vi "Check.vi"(8 "error in (no error)":errorcluster, 11 "Blacklist in":refnum<class "Blacklist.lvclass">) -> (0 "error out":errorcluster, 1 "Reject?":bool, 2 "Output":string, 3 "Blacklist out":refnum<class "Blacklist.lvclass">)   [LabVIEW 2014, in "BuildSecurity.lvlib" / "Blacklist.lvclass"]
doc: "Checks if a VI contains a blacklisted item. If an item is found, <b>Reject?</b> will return <b>TRUE</b>."
uses:
  Blacklist.lvclass
  <vilib>/Utility/traverseref.llb/TRef TravTarget.ctl
  Blacklist.lvclass/Blacklist.ctl
  <vilib>/Utility/traverseref.llb/VI Scripting - Traverse.lvlib
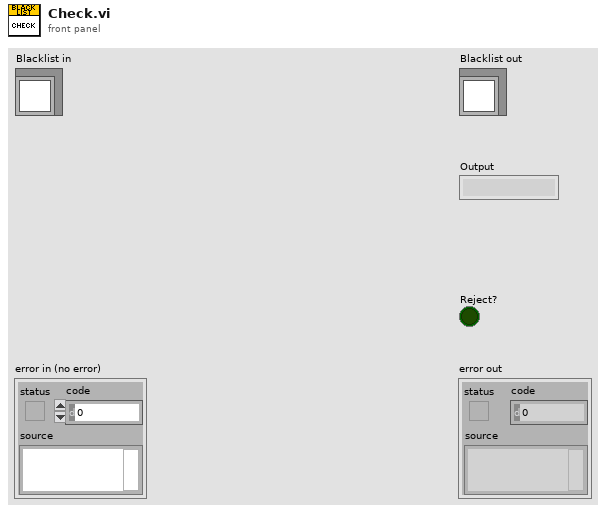
[diagram p1: front panel]
types:
  T1 = typedef "TRef TravTarget.ctl" = enum16{"FP", "BD", "Other"}
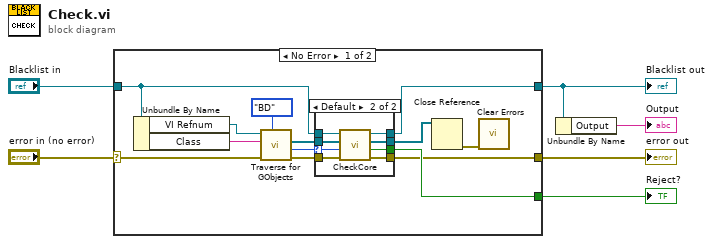
[diagram p0: block diagram]
diagram:
  n1 = case shown="No Error" "error in (no error)" {
    selector: "error in (no error)" -> [w18 w32]
    tunnel: [w7 w32] -> w5
    tunnel: [w11 w31] -> w2
    tunnel: "Blacklist in" -> [w12 w31]
    tunnel: [w9 _] -> w3
    frame No Error {
      n2 = Unbundle By Name(w12) -> ("VI Refnum"=w16:refnum<vi>, "Class"=w19:string)
      n3 = call <vilib>:"Traverse for GObjects.vi"("Traverse Target"=TRef_TravTarget."BD", "error in (no error)"=w18, "Class Name"=w19, "VI Refnum"=w16) -> ("error out"=w14:errorcluster, "# of Refs"=w15:i32, "References"=w13:refnum<vi>[])  [unwired: 4 in, 1 out]
      n4 = case shown="Default" w15 {
        selector: w15 -> [_ w27]
        tunnel: w14 -> [w20 w30]
        tunnel: w13 -> [w21 w28]
        tunnel: w12 -> [w22 w29]
        tunnel: [w22 w26] -> w11
        tunnel: [w21 w25] -> w10
        tunnel: [_ w24] -> w9
        tunnel: [w20 w23] -> w7
        frame 0 {
        }
        frame Default {
          n5 = call-dynamic "CheckCore.vi"("error in (no error)"=w30, "# of Refs"=w27, "References"=w28, "Blacklist in"=w29) -> ("error out"=w23:errorcluster, "Reject?"=w24:bool, "dup References"=w25:refnum<vi>[], "Blacklist out"=w26:refnum<class "Blacklist.lvclass">)  [unwired: 4 in]
        }
      }
      n6 = Close Reference(reference=w10) -> (error out=w8:errorcluster)  [unwired: 1 in]
      n7 = call <vilib>:"Clear Errors.vi"("error in (no error)"=w8) -> ()  [unwired: 5 in, 2 out]
    }
    frame Error {
    }
  }
  "error out" <- w5
  "Blacklist out" <- w2
  "Reject?" <- w3
  n8 = Unbundle By Name(w2) -> ("Output"=→"Output":string)
